vi "platform2Channel_Analog.vi"(9 "mazeDirection":string, 11 "platforms":i32[](array[numeric])) -> (3 "DAQmx Channel":string)   [LabVIEW 2017]
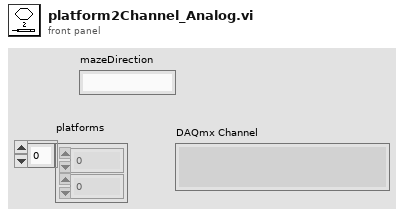
[diagram p1: front panel]
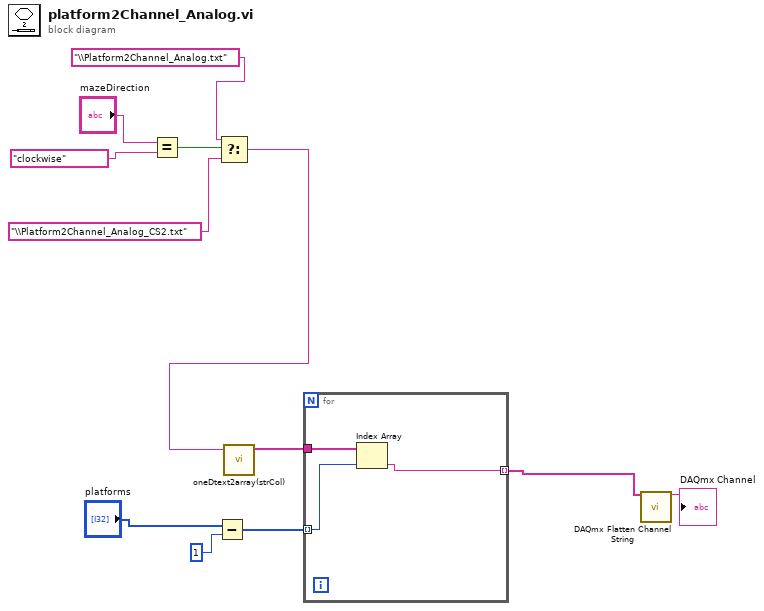
[diagram p0: block diagram]
diagram:
  n1 = Equal?(x="mazeDirection", y="clockwise") -> (x = y?=w4:bool)
  n2 = Subtract(x="platforms", y=1) -> (x-y=w9:i32[])
  n3 = Select(t="\\Platform2Channel_Analog.txt" ("String"), s=w4, f="\\Platform2Channel_Analog_CS2.txt" ("String")) -> (s? t:f=w1:string)
  n4 = call "oneDtext2array(strCol).vi"("String"=w1) -> ("text"=w12:string[])  [unwired: 10 in]
  n5 = for {
    tunnel: w12 -> [w15]
    tunnel: w9 -> [w14] mode=indexing
    tunnel: [w13] -> w8 mode=indexing
    n6 = Index Array(array=w15, index=w14) -> (element=w13:string)
  }
  n7 = call <vilib>:"DAQmx Flatten Channel String.vi"("names in"=w8) -> ("names out"=→"DAQmx Channel":string)  [unwired: 13 in, 1 out]
